vi "TestEMSABandCalculation.vi"() -> ()   [LabVIEW 2017]
uses:
  <vilib>/addons/InsightCM/Devices/Shared/Emsa/EmsaAnalysis/controls/sweepInfo.ctl
  <vilib>/addons/InsightCM/Devices/Shared/Emsa/EmsaAnalysis/EmsaAnalysis.lvlib
panel:
  out "power in band":dbl format="%#_4p"
  in  "stop frequency":dbl=-1.0 format="%#_6p"
  in  "start frequency":dbl=-1.0 format="%#_6p"
  out "combined power in band":dbl=0.00018833215658045667 format="%#_3p"
  out "power in band 2":dbl=7.379548729079718e-05 format="%#_3p"
  out "power in band 1":dbl=0.000173272119101024 format="%#_3p"
  in  "start frequency 2":dbl=750000.0 format="%#_3p"
  in  "stop frequency 2":dbl=1000000.0 format="%#_3p"
  in  "stop frequency 1":dbl=750000.0 format="%#_3p"
  in  "start frequency 1":dbl=400000.0 format="%#_3p"
  in  "bandwidth":dbl=9000.0 format="%#_13g"
  out "Channel Voltage":dbl=0.00018823344918322422 format="%#_3p"
  in  "index 4":i32=1
  in  "Power Stop Freq":dbl=1000000.0 format="%#_6p"
  in  "Power Start Freq":dbl=400000.0 format="%#_6p"
  in  "index 3":i32=4
  out "XY Graph 3":cluster{dbl[], "Filtered X":dbl[]}[](graph)
  out "XY Graph 2":cluster{dbl[], dbl[]}[](graph)
  in  "index 2":i32=3
  in  "stop":bool
  in  "path":path=path "C:/Users/Administrator/Desktop/Hines EMSA/Hines EMSA/PB1-PNL-EMSA-1B-01/2015/09"
  out "XY Graph":cluster{dbl[], dbl[]}[](graph)
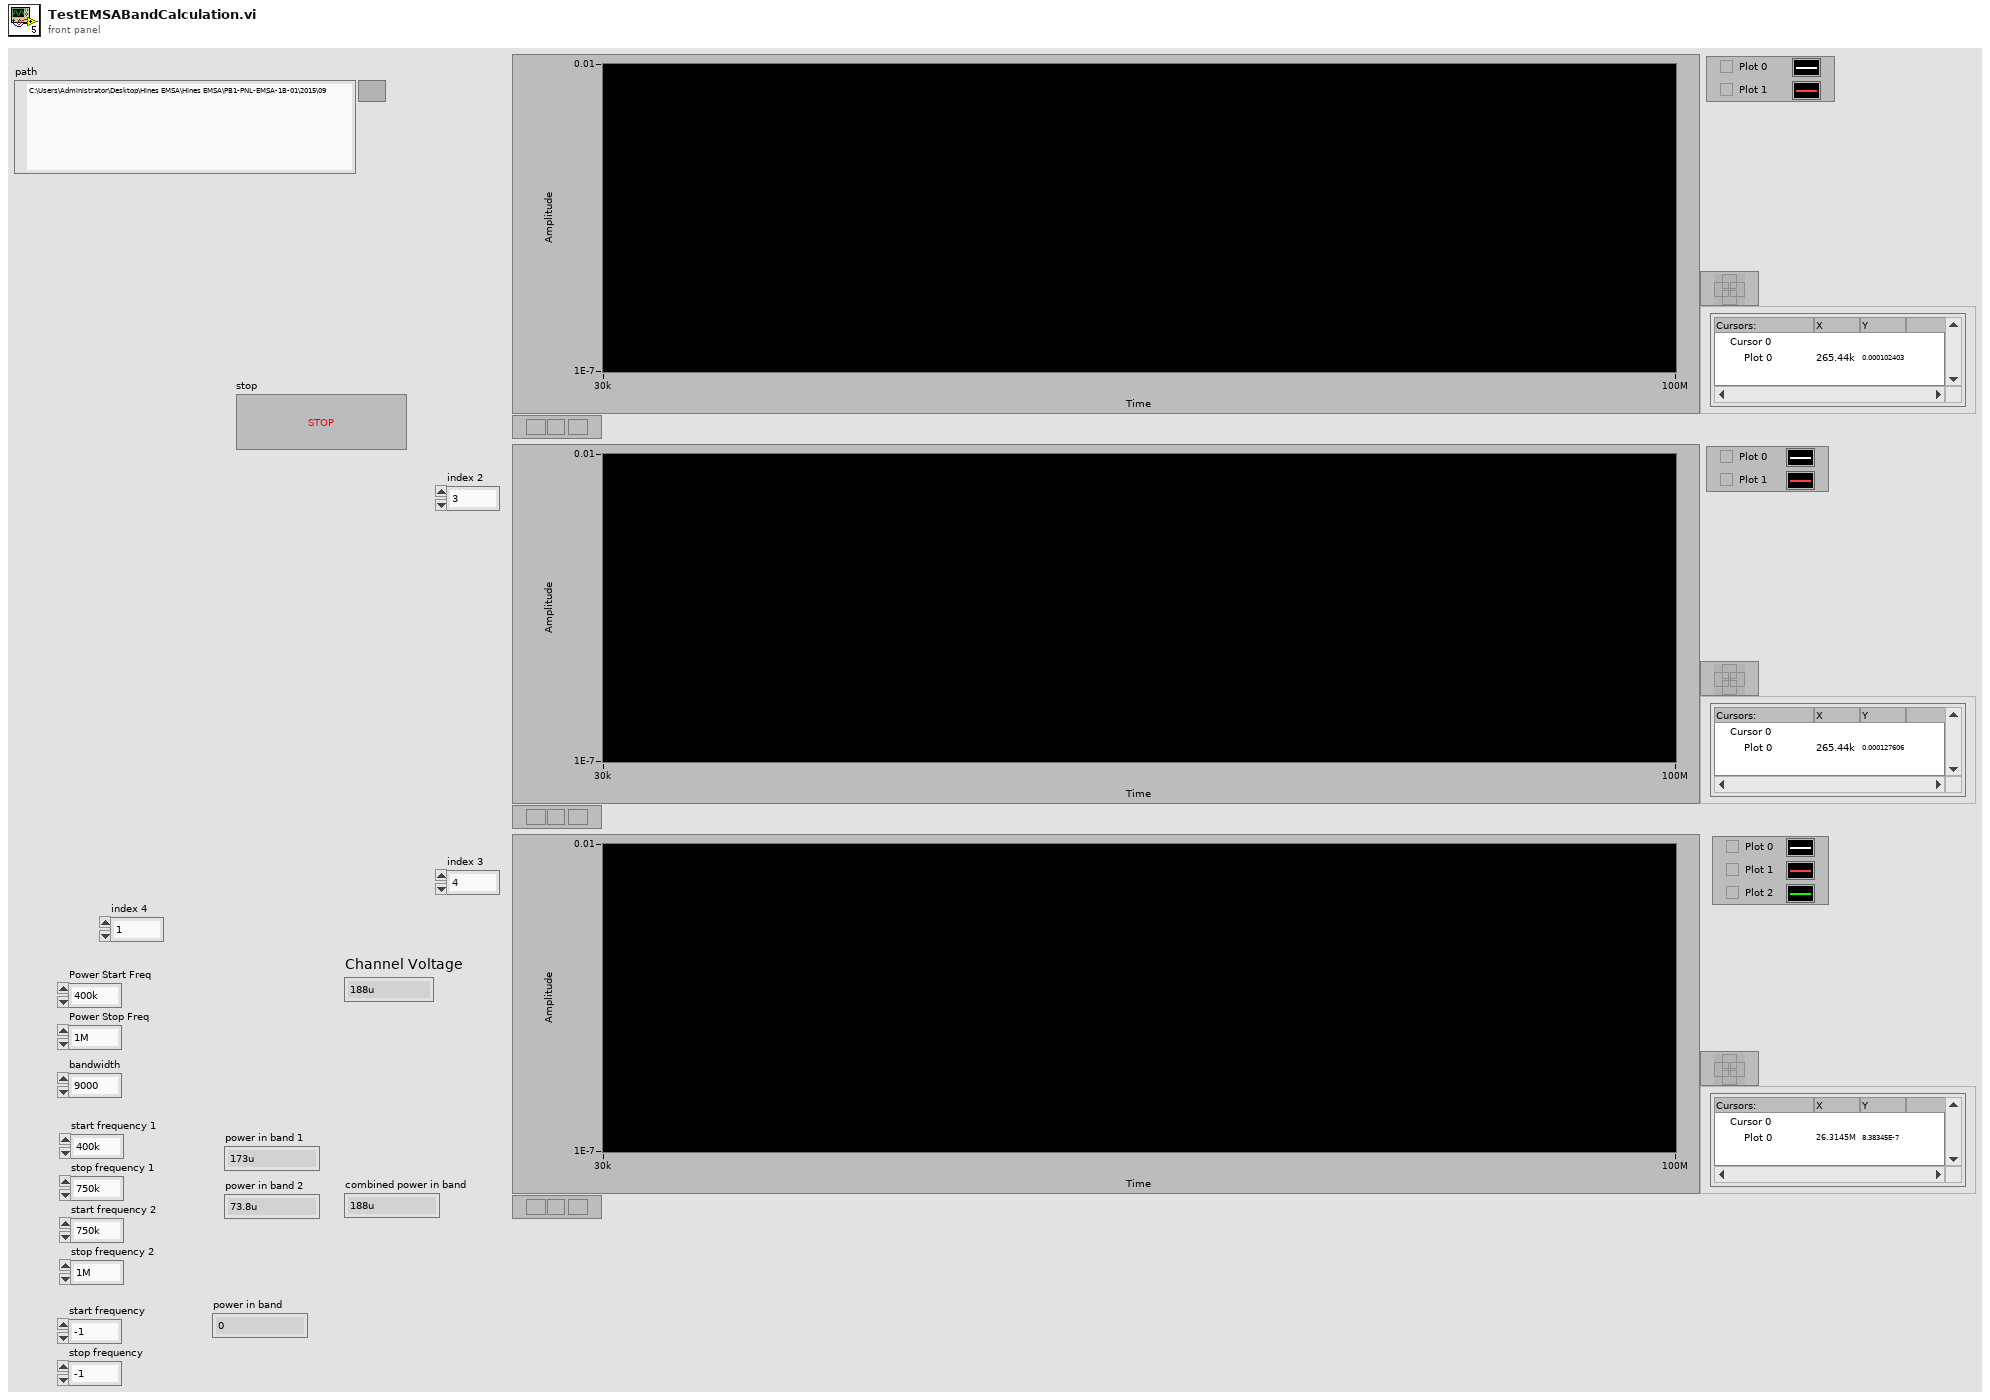
[diagram p1: front panel]
types:
  T1 = typedef "EMSAAnalysis.lvlib/sweepInfo.ctl" = cluster{"start":dbl, "stop":dbl, "bandwidth":dbl}
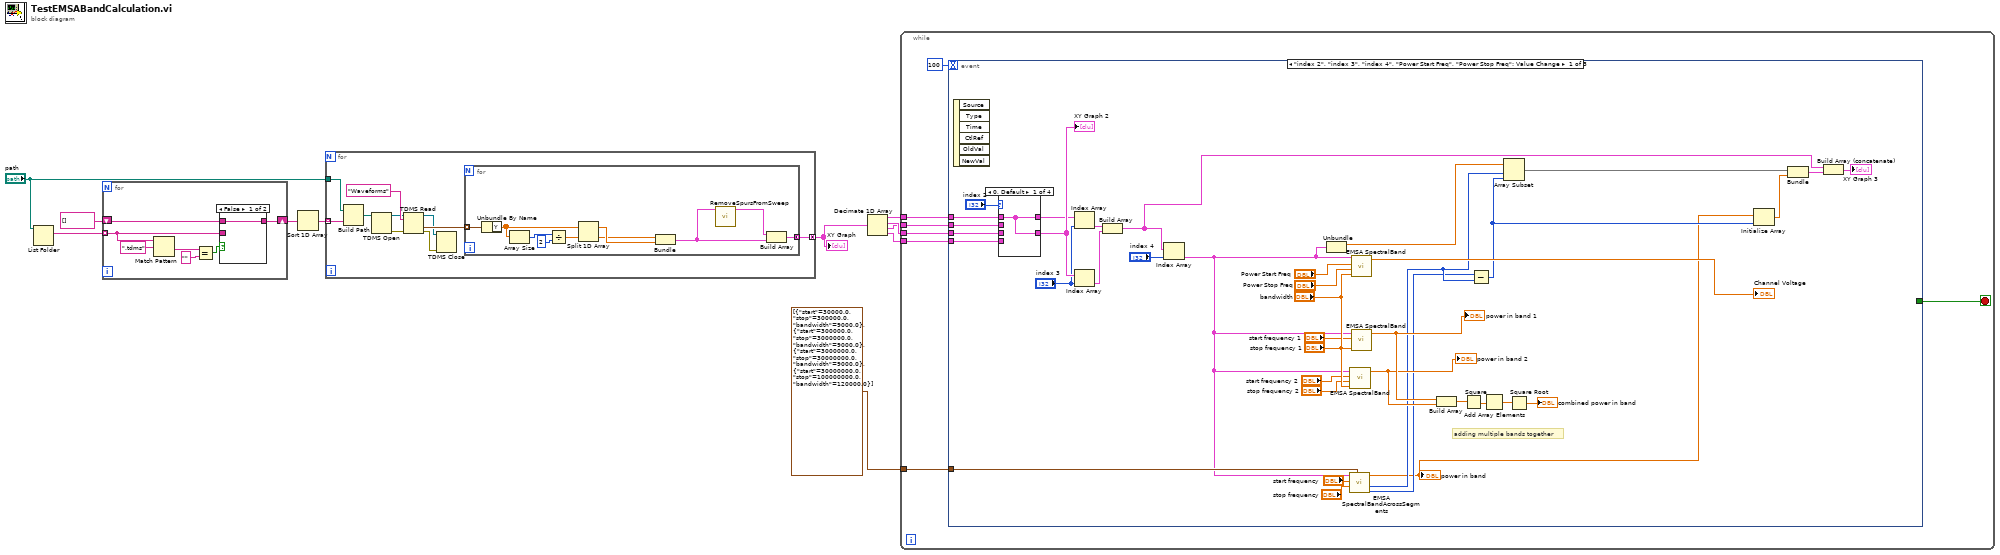
[diagram p0: block diagram]
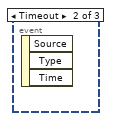
[diagram p5: hidden frame]
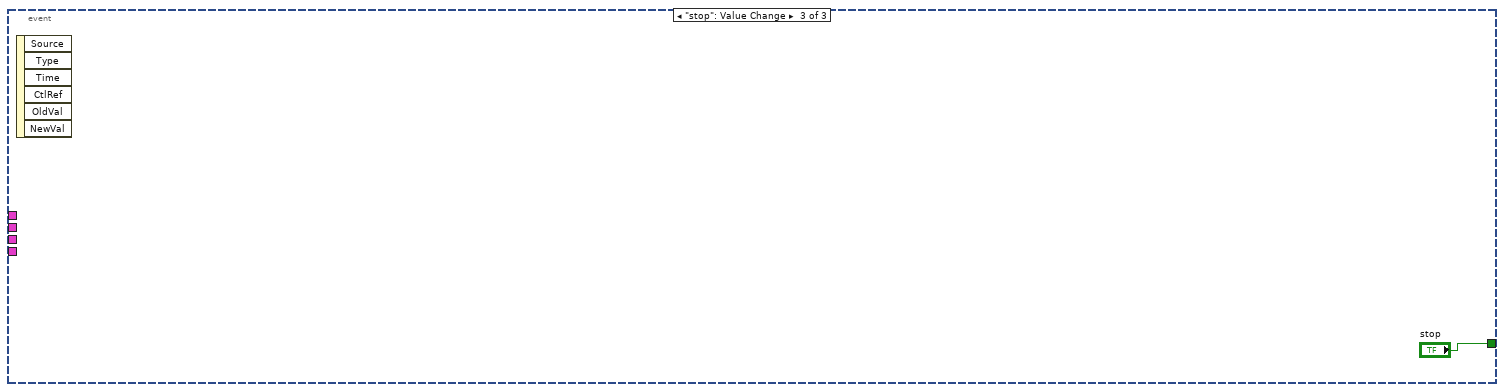
[diagram p6: hidden frame]
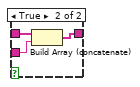
[diagram p7: hidden frame]
diagram:
  n1 = List Folder(path="path") -> (filenames=w11:string[])  [unwired: 3 in, 3 out]
  n2 = for {
    tunnel: w11 -> [w15] mode=indexing
    shift-right: [w14] -> w6
    shift-left: string[] [] -> [w13]
    n3 = Match Pattern(string=w15, regular expression=".tdms") -> (after substring=w17:string)  [unwired: 1 in, 3 out]
    n4 = Equal?(x=w17, y="") -> (x = y?=w12:bool)
    n5 = case shown="False" w12 {
      tunnel: w15 -> [_ w22]
      tunnel: [w19 w21] -> w14
      tunnel: w13 -> [w19 w20]
      frame False {
      }
      frame True {
        n6 = Build Array (concatenate)(w20, w22) -> (w21:string[])
      }
    }
  }
  n7 = Sort 1D Array(array=w6) -> (sorted array=w5:string[])
  n8 = for {
    tunnel: w5 -> [w32] mode=indexing
    tunnel: "path" -> [w31]
    tunnel: [w23] -> w9 mode=concatenating
    n9 = Build Path(base path=w31, name or relative path=w32) -> (appended path=w24:path)
    n10 = TDMS Open(11:w24) -> (0:w26:errorcluster, 3:w25:refnum<k34>)  [unwired: 6 in]
    n11 = TDMS Read(0:w25, 5:"Waveforms" ("group name in"), 11:w26) -> (4:w29:refnum<k34>, 10:w30:waveform(dbl)[], 15:w28:errorcluster)  [unwired: 5 in, 3 out]
    n12 = TDMS Close(8:w28, 11:w29) -> ()  [unwired: 2 out]
    n13 = for {
      tunnel: w30 -> [w42] mode=indexing
      tunnel: [w36] -> w23 mode=concatenating
      n14 = Unbundle By Name(w42) -> ("Y"=w41:dbl[])
      n15 = Array Size(array=w41) -> (size(s)=w38:i32)
      n16 = Divide(x=w38, y=2) -> (x/y=w39:dbl)
      n17 = Split 1D Array(array=w41, index=w39) -> (first subarray=w37:dbl[], second subarray=w35:dbl[])
      n18 = Bundle(w35, w37) -> (w34:cluster{dbl[], dbl[]})  [unwired: 1 in]
      n19 = call <vilib>:"RemoveSpursFromSweep.vi"("sweep"=w34) -> ("sweep"=w33:cluster{"frequency":dbl[], "amplitude":dbl[]})  [unwired: 10 in]
      n20 = Build Array(w33, w34) -> (w36:cluster{"frequency":dbl[], "amplitude":dbl[]}[])
    }
  }
  "XY Graph" <- w9
  n21 = Decimate 1D Array(w9) -> (w8:cluster{"frequency":dbl[], "amplitude":dbl[]}[], w4:cluster{"frequency":dbl[], "amplitude":dbl[]}[], w3:cluster{"frequency":dbl[], "amplitude":dbl[]}[], w2:cluster{"frequency":dbl[], "amplitude":dbl[]}[])
  n22 = while {
    tunnel: w8 -> [w49]
    tunnel: w4 -> [w48]
    tunnel: w3 -> [w47]
    tunnel: w2 -> [w46]
    tunnel: T1[] [{"start"=30000.0, "stop"=300000.0, "bandwidth"=9000.0}, {"start"=300000.0, "stop"=3000000.0, "bandwidth"=9000.0}, {"start"=3000000.0, "stop"=30000000.0, "bandwidth"=9000.0}, {"start"=30000000.0, "stop"=100000000.0, "bandwidth"=120000.0}] ("sweeps") -> [w43]
    stop <- w44 stop-if-true
    n23 = event shown="[0] \"index 2\", \"index 3\", \"index 4\", \"Power Start Freq\", \"Power Stop Freq\": Value Change" {
      selector: _ -> [_ _ _]
      dyn-events: _ -> [_ _ _]
      timeout: 100 -> [_ _ _]
      tunnel: w49 -> [w87 _ _]
      tunnel: w48 -> [w86 _ _]
      tunnel: w47 -> [w85 _ _]
      tunnel: w46 -> [w84 _ _]
      tunnel: [_ _ "stop"] -> w44
      tunnel: w43 -> [w56 _ _]
      event "index 2", "index 3", "index 4", "Power Start Freq", "Power Stop Freq": Value Change {
        # "adding multiple bands together"
        n24 = event-data() -> ()  [unwired: 1 in, 6 out]
        n25 = case shown="0, Default" "index 2" {
          tunnel: w87 -> [w89 w90 _ _]
          tunnel: [w89 w91 w92 w94] -> w83
          tunnel: w86 -> [_ w91 _ _]
          tunnel: w85 -> [_ _ w92 w93]
          tunnel: w84 -> [_ _ _ w94]
          tunnel: [w89 w90 w92 w93] -> w82
          frame 0, Default {
          }
          frame 1 {
          }
          frame 2 {
          }
          frame 3 {
          }
        }
        "XY Graph 2" <- w83
        n26 = Index Array(array=w82, index="index 3") -> (element=w80:cluster{"frequency":dbl[], "amplitude":dbl[]})
        n27 = Index Array(array=w83, index="index 3") -> (element=w79:cluster{"frequency":dbl[], "amplitude":dbl[]})
        n28 = Build Array(w80, w79) -> (w77:cluster{"frequency":dbl[], "amplitude":dbl[]}[])
        n29 = Index Array(array=w77, index="index 4") -> (element=w55:cluster{"frequency":dbl[], "amplitude":dbl[]})
        n30 = Unbundle(w55) -> ("frequency"=w71:dbl[])  [unwired: 1 out]
        n31 = call <vilib>:"EMSA SpectralBandAcrossSegments.vi"("sweeps"=w56, "stop frequency"="stop frequency", "start frequency"="start frequency", "sweep in"=w55) -> ("stop index"=w51:i32, "start index"=w52:i32, "power in band"=w50:dbl)  [unwired: 5 in]
        "power in band" <- w50
        n32 = call <vilib>:"EMSA SpectralBand.vi"("bandwidth"="bandwidth", "stop frequency"="stop frequency 2", "start frequency"="start frequency 2", "sweep in"=w55) -> ("power in band"=w57:dbl)  [unwired: 5 in, 2 out]
        "power in band 2" <- w57
        n33 = call <vilib>:"EMSA SpectralBand.vi"("bandwidth"="bandwidth", "stop frequency"="Power Stop Freq", "start frequency"="Power Start Freq", "sweep in"=w55) -> ("power in band"=→"Channel Voltage":dbl)  [unwired: 5 in, 2 out]
        n34 = call <vilib>:"EMSA SpectralBand.vi"("bandwidth"="bandwidth", "stop frequency"="stop frequency 1", "start frequency"="start frequency 1", "sweep in"=w55) -> ("power in band"=w58:dbl)  [unwired: 5 in, 2 out]
        "power in band 1" <- w58
        n35 = Build Array(w58, w57) -> (w62:dbl[])
        n36 = Square(x=w62) -> (x^2=w61:dbl[])
        n37 = Subtract(x=w51, y=w52) -> (x-y=w69:i32)
        n38 = Add Array Elements(numeric array=w61) -> (sum=w60:dbl)
        n39 = Array Subset(array=w71, index=w52, length=w69) -> (w75:dbl[])
        n40 = Square Root(x=w60) -> (sqrt(x)=→"combined power in band":dbl)
        n41 = Initialize Array(w50, w69) -> (w74:dbl[])
        n42 = Bundle(w75, w74) -> (w68:cluster{dbl[], dbl[]})  [unwired: 1 in]
        n43 = Build Array (concatenate)(w77, w68) -> (→"XY Graph 3":cluster{"frequency":dbl[], "amplitude":dbl[]}[])
      }
      event Timeout {
        n44 = event-data() -> ()  [unwired: 1 in, 3 out]
      }
      event "stop": Value Change {
        n45 = event-data() -> ()  [unwired: 1 in, 6 out]
      }
    }
  }
